vi "程序设置-删除程序.vi"() -> (2 "程序号输出":i32, 3 "Cancelled?":bool caption="取消？")   [LabVIEW 2014]
doc: "该模板用于创建能够进行事件处理的对话框。"
panel:
  out "错误输出":errorcluster
  in  "™C·Nßx“ñ":i32(ring) items=["程序0-----000"]
  in  "Cancel":bool caption="取消"
  in  "OK":bool caption="确定"
  # "删除程序"
  # "选择要删除程序:"
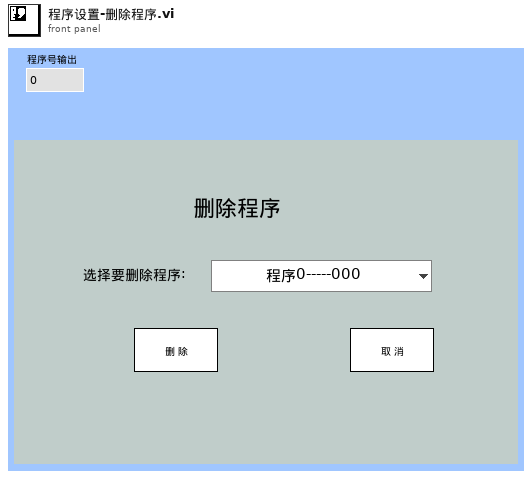
[diagram p1: front panel]
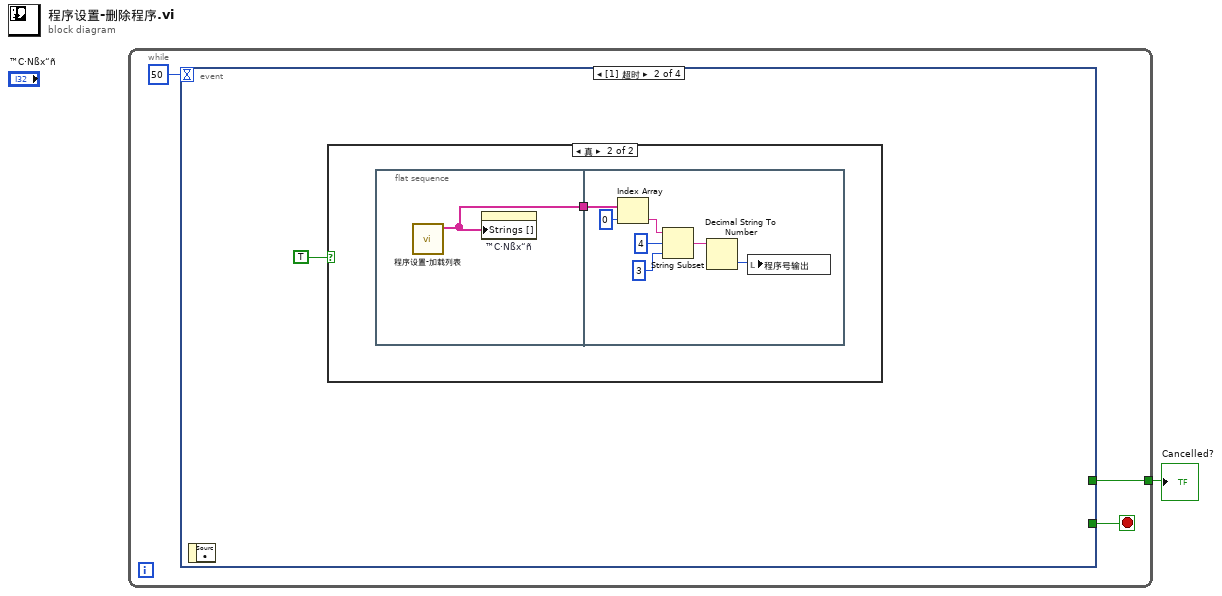
[diagram p0: block diagram]
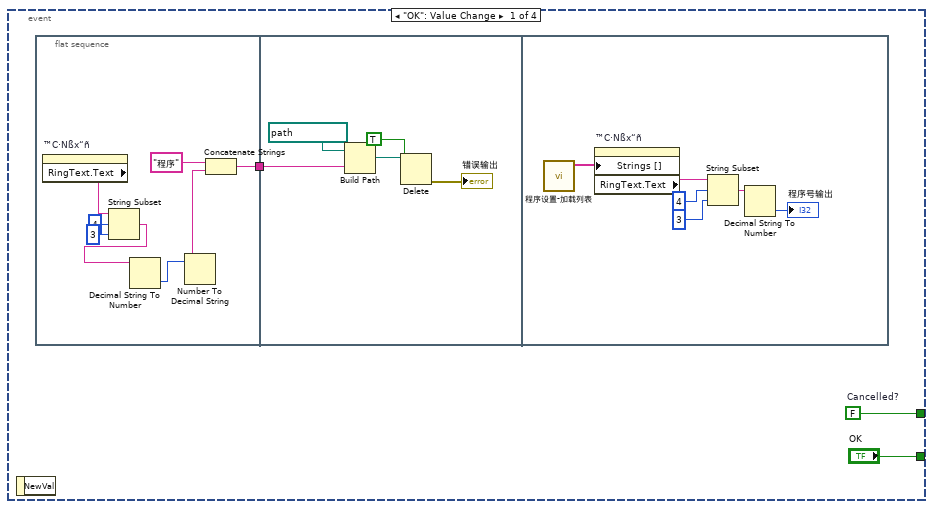
[diagram p2: hidden frame]
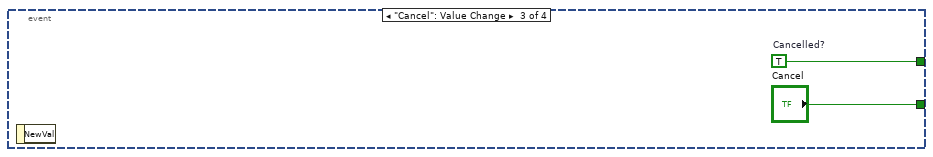
[diagram p4: hidden frame]
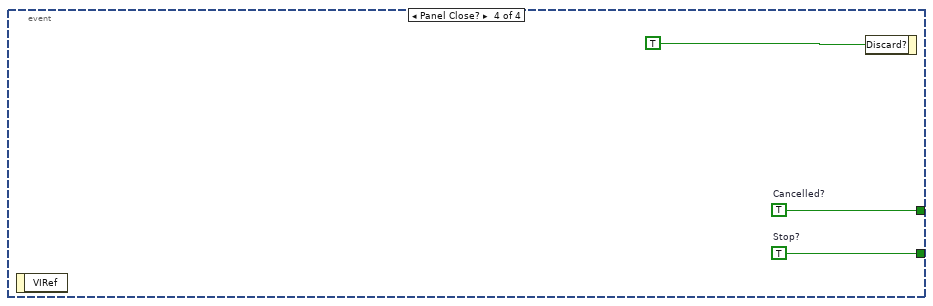
[diagram p5: hidden frame]
diagram:
  n1 = while {
    tunnel: [w3] -> w1
    stop <- w4 stop-if-true
    n2 = event shown="[1] 超时" {
      selector: _ -> [_ _ _ _]
      dyn-events: _ -> [_ _ _ _]
      timeout: 50 -> [_ _ _ _]
      tunnel: ["OK" _ "Cancel" w40] -> w4
      tunnel: [w7 _ w38 w39] -> w3
      event "OK": Value Change {
        w7 = FALSE  # Cancelled?
        n3 = event-data() -> ()  [unwired: 1 in, 1 out]
        n4 = flat-sequence {
          tunnel: [w13] -> w5
          tunnel: w5 -> [w17]
          frame #0 {
            n5 = property on="™C·Nßx“ñ" class="Ring (严格)"() -> ("RingText.Text"=w15:string)  [unwired: 2 in, 2 out]
            n6 = String Subset(string=w15, offset (0)=4 ("偏移量(0)"), length (rest)=3 ("长度（剩余）")) -> (substring=w12:string)
            n7 = Decimal String To Number(string=w12) -> (number=w11:i32)  [unwired: 2 in, 1 out]
            n8 = Number To Decimal String(number=w11) -> (decimal integer string=w10:string)  [unwired: 1 in]
            n9 = Concatenate Strings("程序" ("字符串"), w10) -> (w13:string)
          }
          frame #1 {
            n10 = Build Path(base path=path "D:/程序参数" ("基路径"), name or relative path=w17) -> (appended path=w19:path)
            n11 = Delete(path (use dialog)=w19, entire hierarchy (F)=TRUE ("整个层次结构(F)")) -> (error out=→"错误输出":errorcluster)  [unwired: 3 in, 2 out]
          }
          frame #2 {
            n12 = call "程序设置-加载列表.vi"() -> ("文件名显示"=w22:string[])  [unwired: 10 in, 1 out]
            n13 = property on="™C·Nßx“ñ" class="Ring (严格)"("Strings []"=w22) -> ("RingText.Text"=w21:string)  [unwired: 2 in, 2 out]
            n14 = String Subset(string=w21, offset (0)=4 ("偏移量(0)"), length (rest)=3 ("长度（剩余）")) -> (substring=w26:string)
            n15 = Decimal String To Number(string=w26) -> (number=→"程序号输出":i32)  [unwired: 2 in, 1 out]
          }
        }
      }
      event Timeout {
        n16 = event-data() -> ()  [unwired: 1 in, 1 out]
        n17 = case shown="真" TRUE {
          frame False {
          }
          frame True {
            n18 = flat-sequence {
              tunnel: [w29] -> w28
              tunnel: w28 -> [w32]
              frame #0 {
                n19 = call "程序设置-加载列表.vi"() -> ("文件名显示"=w29:string[])  [unwired: 10 in, 1 out]
                n20 = property on="™C·Nßx“ñ" class="Ring (严格)"("Strings []"=w29) -> ()  [unwired: 2 in, 2 out]
              }
              frame #1 {
                n21 = Index Array(array=w32, index=0 ("索引")) -> (element=w30:string)
                n22 = String Subset(string=w30, offset (0)=4 ("偏移量(0)"), length (rest)=3 ("长度（剩余）")) -> (substring=w34:string)
                n23 = Decimal String To Number(string=w34) -> (number=w33:i32)  [unwired: 2 in, 1 out]
                n24 = local write "程序号输出"(w33) -> ()
              }
            }
          }
        }
      }
      event "Cancel": Value Change {
        w38 = TRUE  # Cancelled?
        n25 = event-data() -> ()  [unwired: 1 in, 1 out]
      }
      event Panel Close? {
        w39 = TRUE  # Cancelled?
        w40 = TRUE  # Stop?
        n26 = event-data() -> ()  [unwired: 1 in, 1 out]
        n27 = event-data("Discard?"=TRUE) -> ()  [unwired: 1 in, 1 out]
      }
    }
  }
  "Cancelled?" <- w1
